vi "Autonomous Independent.vi"() -> ()   [LabVIEW 2015]
doc: "This VI is called when autonomous begins, and will automatically be terminated when autonomous ends. You can carry out timed or sensor driven robot movement independently without needing to return to the caller."
uses:
  <vilib>/Rock Robotics/WPI/CAN/TalonSRX/WPI_CANTalonSRX_BrakeOverride.ctl
  <vilib>/Rock Robotics/WPI/Solenoid/WPI_SolenoidValue.ctl
  <vilib>/Analysis/baseanly.llb/Mean (DBL).vi
  <vilib>/Rock Robotics/WPI/Utilities/WPI_GetSetVariantRefNum.vi
  <vilib>/Rock Robotics/Network Tables/NT Write Numeric Array.vi
  <vilib>/Rock Robotics/Network Tables/NT Read Numeric Array.vi
  <vilib>/Rock Robotics/Network Tables/NT Read String Array.vi
  <vilib>/Rock Robotics/Network Tables/NT Write String.vi
  <vilib>/addons/control/pid/pid.llb/PID (DBL).vi
  <vilib>/Rock Robotics/WPI/Solenoid/WPI_SolenoidSetEnum.vi
  ADI MXP IMU/ADI MXP IMU/FRC ADI MXP IMU.lvlib
  <vilib>/addons/control/pid/NI_PID_pid.lvlib
  <vilib>/Analysis/NI_AALBase.lvlib
panel:
  out "Waveform Chart":dbl(graph)
  out "Rotate PID Output":dbl(graph)
  # "Be sure to right-click and choose Data Operations>>Make Current Value default if you want to save the array values with the VI"
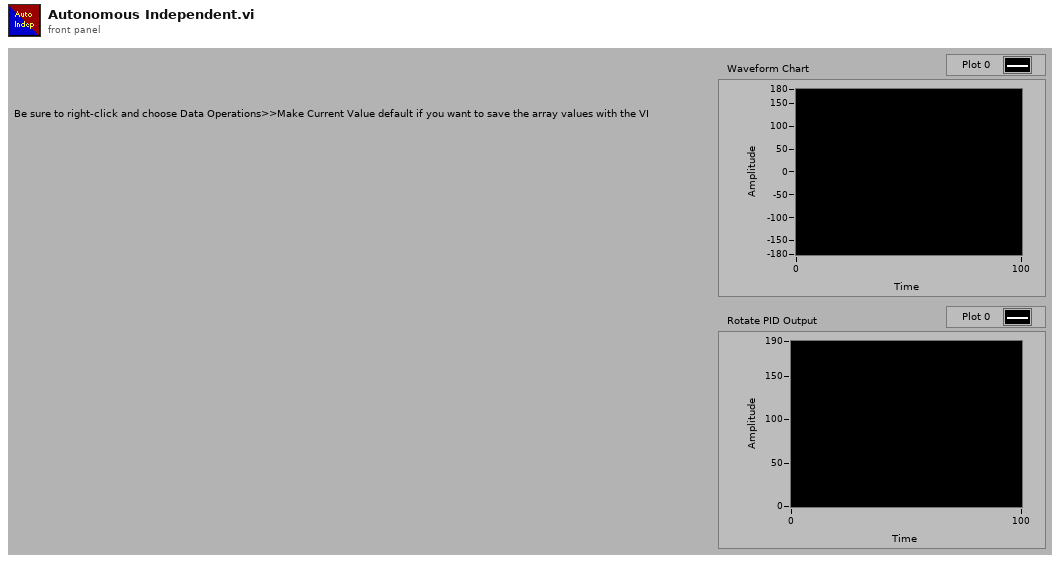
[diagram p1: front panel]
types:
  T1 = typedef "WPI_EncoderDevRef.ctl" = cluster{"DevStatus":errorcluster, "EncoderIndex":T2, "CounterIndex":T3, "DistancePerCount":dbl, "Decoding Type":T4}
  T2 = typedef "FPGA_EncoderIdx.ctl" = enum8{"Enc 0", "Enc 1", "Enc 2", "Enc 3", "Enc 4", "Enc 5", "Enc 6", "Enc 7", "Invalid"}
  T3 = typedef "FPGA_CounterCtrSystemIndex.ctl" = enum8{"Ctr 0", "Ctr 1", "Ctr 2", "Ctr 3", "Ctr 4", "Ctr 5", "Ctr 6", "Ctr 7", "Invalid"}
  T4 = typedef "WPI_EncoderType.ctl" = enum16{"1x", "2x", "4x"}
  T5 = cluster{"proportional gain (Kc)":dbl, "integral time (Ti, min)":dbl, "derivative time (Td, min)":dbl}
  T6 = typedef "WPI_SolenoidValue.ctl" = enum16{"Off", "On", "Forward", "Reverse"}
  T7 = typedef "WPI_CANTalonSRX_BrakeOverride.ctl" = enum8{"No Override", "Override to Coast", "Override to Brake"}
  T8 = typedef "FRC ADI MXP IMU.lvlib/WPI_AnalogDevicesIMUInterruptDevRef.ctl" = cluster{"SimpleGyroDevRef":T9, "InterruptRef":T11}
  T9 = typedef "FRC ADI MXP IMU.lvlib/WPI_AnalogDevicesIMUDevRef.ctl" = cluster{"DevStatus":errorcluster, "Handle":i32, "SPI Bus":T10, "Device Found":bool, "Sample Rate":dbl, "Device Ready":bool, "Yaw Axis":enum16{"X", "Y", "Z"}, "AHRS Algorithm":enum16{"Complementary", "Madgwick"}}
  T10 = typedef "spi_bus.ctl" = enum16{"SPI On-Board, CS0", "SPI On-Board, CS1", "SPI On-Board, CS2", "SPI On-Board, CS3", "SPI MXP", "Invalid"}
  T11 = typedef "WPI_InterruptRef.ctl" = cluster{"DevStatus":errorcluster, "InterruptIndex":T12}
  T12 = typedef "FPGA_InterruptIndex.ctl" = enum8{"0", "1", "2", "3", "4", "5", "6", "7", "Invalid"}
  T13 = typedef "WPI_SolenoidDevRef.ctl" = cluster{"DevStatus":errorcluster, "Pneumatics Control Module":u8, "Forward Solenoid Channel":T14, "Reverse Solenoid Channel":T14}
  T14 = typedef "WPI_SolenoidChannel.ctl" = enum8{"Solenoid 0", "Solenoid 1", "Solenoid 2", "Solenoid 3", "Solenoid 4", "Solenoid 5", "Solenoid 6", "Solenoid 7", "Invalid"}
  T15 = typedef "WPI_MotorControlDeviceRef.ctl" = cluster{"DeviceStatus":errorcluster, "Type":T16, "PWM":cluster{"PWM Channel":T17, "DeadBand":T18}, "CAN":cluster{"Device Number":u8, "Control Mode":T19, "Semaphore":T20, "Max Vout":dbl, "TalonSRX Control Mode":T21}, "Invert":bool}
  T16 = typedef "WPI_MotorControlType.ctl" = enum16{"PWM", "CAN", "CANTalonSRX"}
  T17 = typedef "FPGA_DIOPWMChannel.ctl" = enum8{"PWM 0", "PWM 1", "PWM 2", "PWM 3", "PWM 4", "PWM 5", "PWM 6", "PWM 7", "PWM 8", "PWM 9", "PWM MXP 0", "PWM MXP 1", "PWM MXP 2", "PWM MXP 3", "PWM MXP 4", "PWM MXP 5", "PWM MXP 6", "PWM MXP 7", "PWM MXP 8", "PWM MXP 9", "Invalid"}
  T18 = typedef "WPI_PWMDeadband.ctl" = cluster{"Name":string, "maxPositivePwm":i32, "minPositivePwm":i32, "centerPwm":i32, "maxNegativePwm":i32, "minNegativePwm":i32, "angularRange":u16}
  T19 = typedef "WPI_CANJaguar_ControlMode.ctl" = enum8{"Percent VBus", "Current", "Speed", "Position", "Voltage"}
  T20 = typedef "Semaphore RefNum" = refnum<k1>
  T21 = typedef "WPI_CANTalonSRX_APIControlMode.ctl" = enum8{"Percent VBus", "Speed", "Position", "Slave", "Unchanged / Invalid", "Voltage Compensation", "Current", "Motion Profile"}
  T22 = typedef "WPI_SwitchDevRef.ctl" = cluster{"DevStatus":errorcluster, "DIO Channel":T23, "CntIndex":T3, "Normally Closed":bool}
  T23 = typedef "FPGA_DIOChannel.ctl" = enum8{"DIO 0", "DIO 1", "DIO 2", "DIO 3", "DIO 4", "DIO 5", "DIO 6", "DIO 7", "DIO 8", "DIO 9", "DIO MXP 0", "DIO MXP 1", "DIO MXP 2", "DIO MXP 3", "DIO MXP 4", "DIO MXP 5", "DIO MXP 6", "DIO MXP 7", "DIO MXP 8", "DIO MXP 9", "DIO MXP 10", "DIO MXP 11", "DIO MXP 12", "DIO MXP 13", "DIO MXP 14", "DIO MXP 15", "Invalid"}
  T24 = cluster{"X Angle":dbl, "Y Angle":dbl, "Z Angle":dbl}
  T25 = typedef "WPI_JoystickDevRef.ctl" = cluster{"Device":T26}
  T26 = typedef "WPI_JoystickDeviceEnum.ctl" = enum16{"USB 0", "USB 1", "USB 2", "USB 3", "USB 4", "USB 5"}
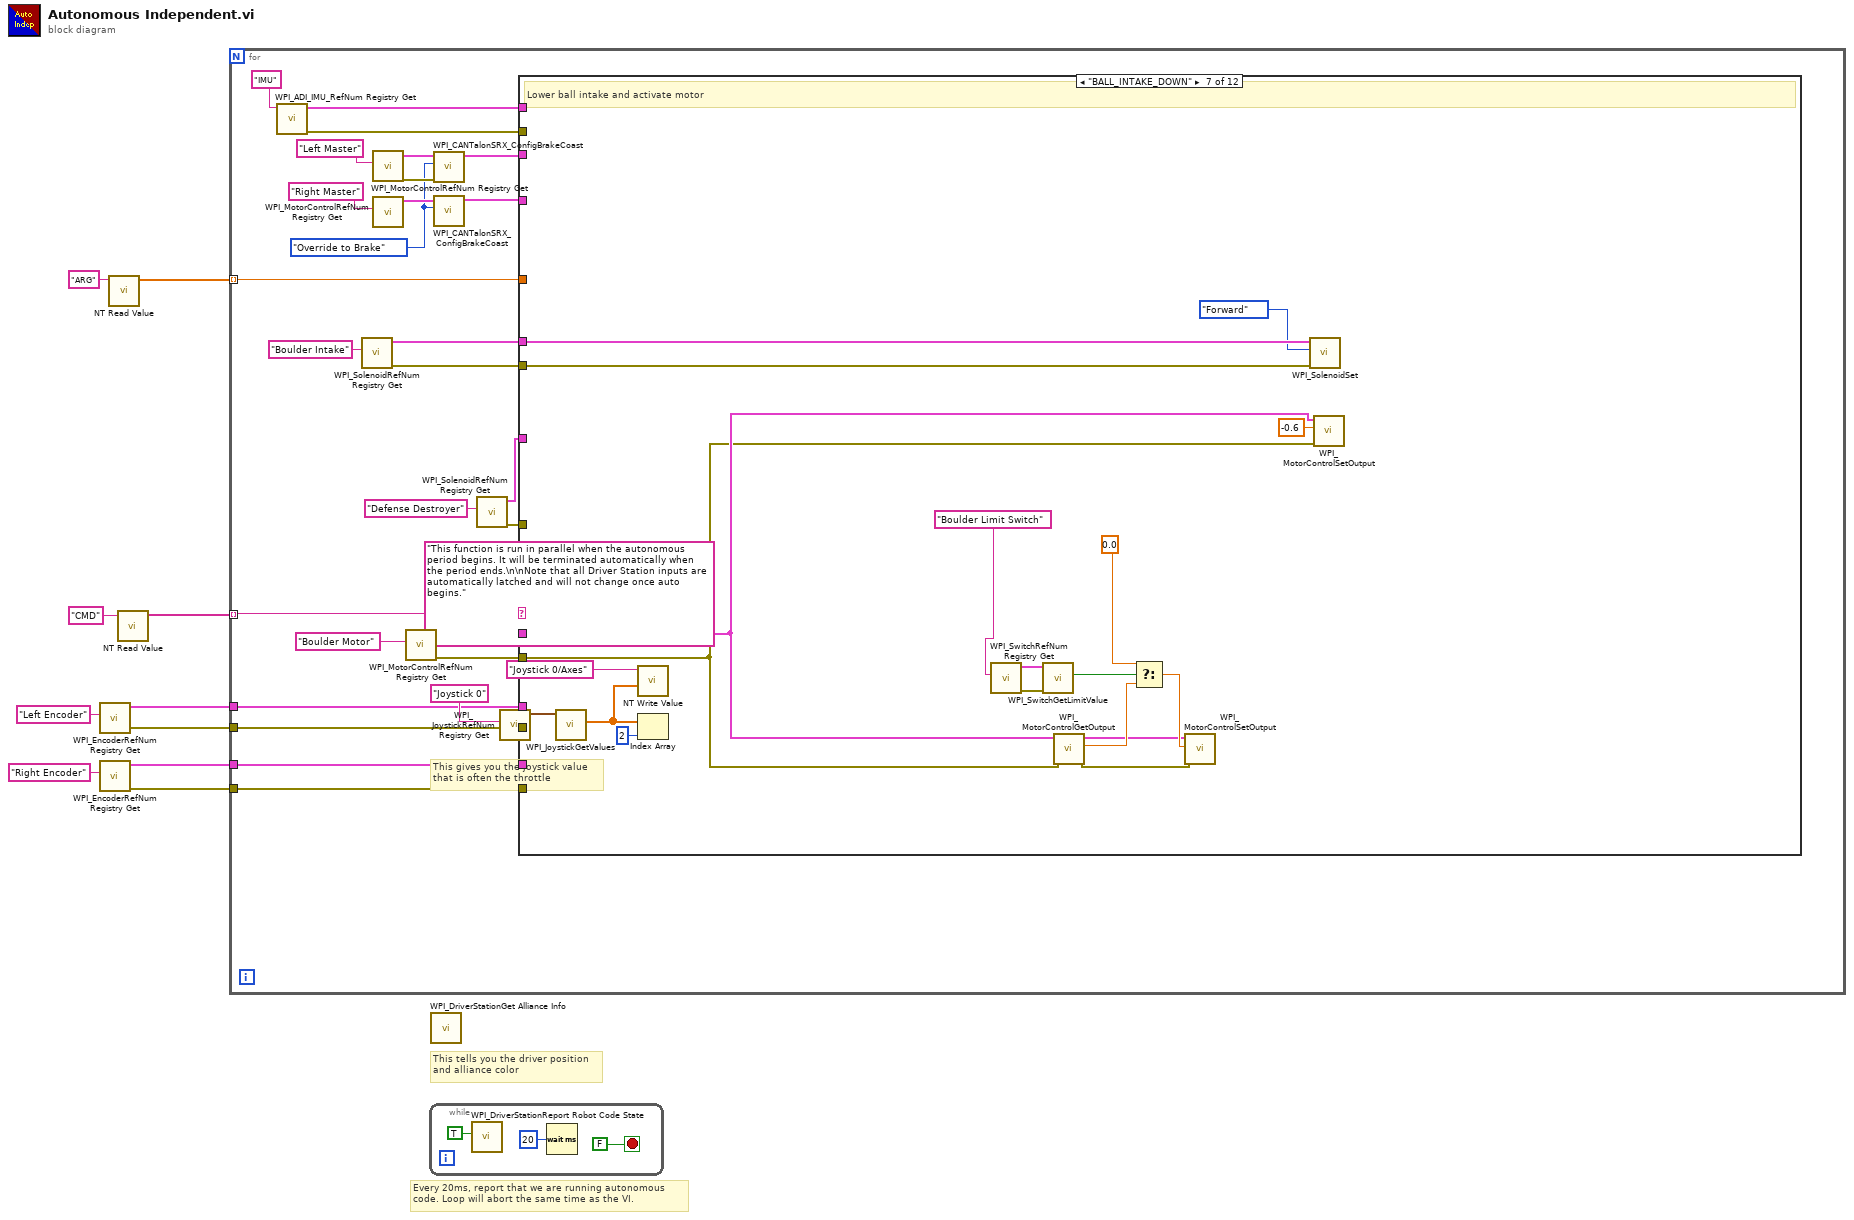
[diagram p0: block diagram]
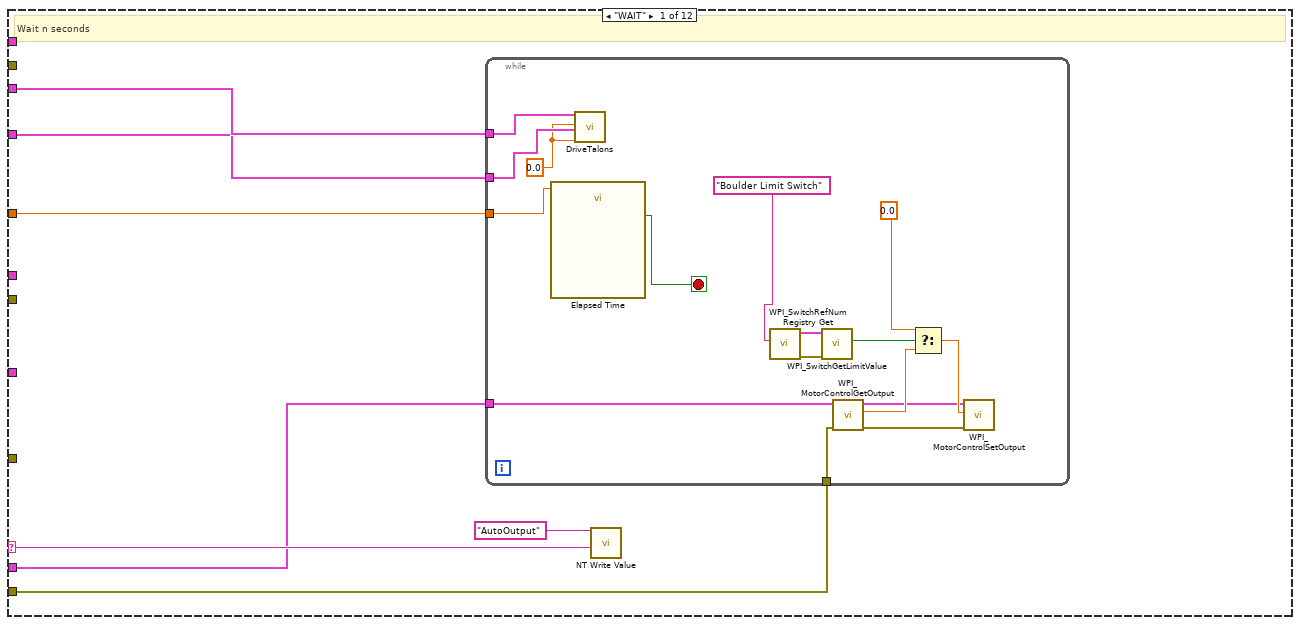
[diagram p2: hidden frame]
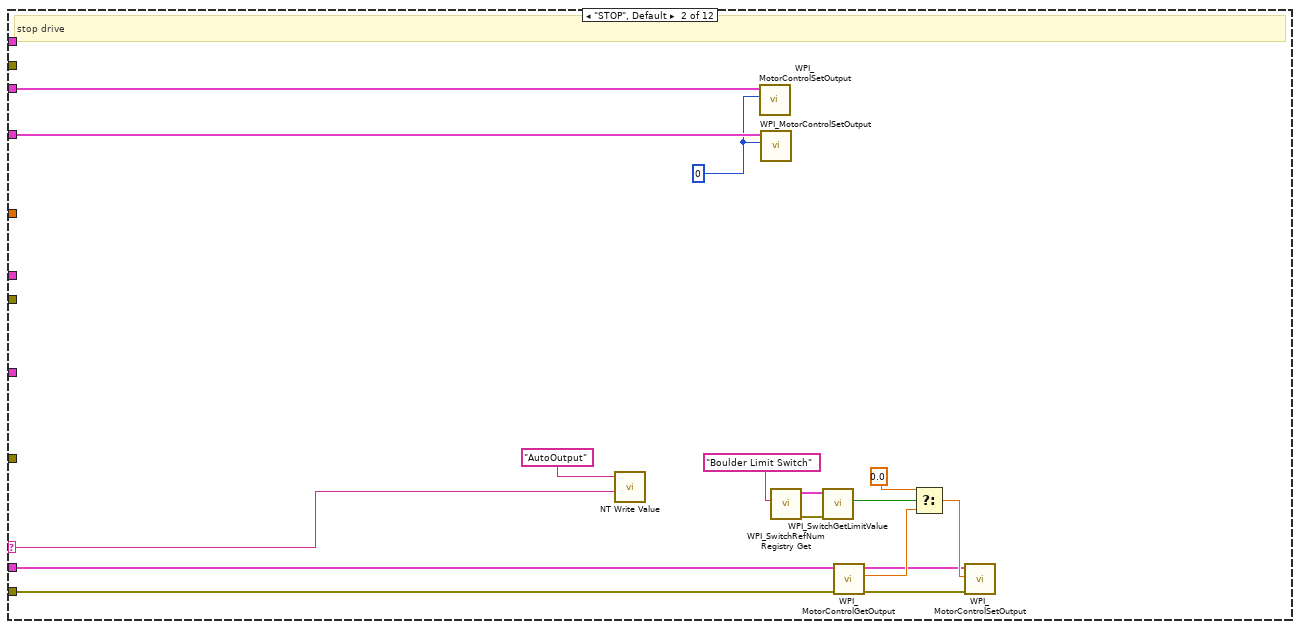
[diagram p3: hidden frame]
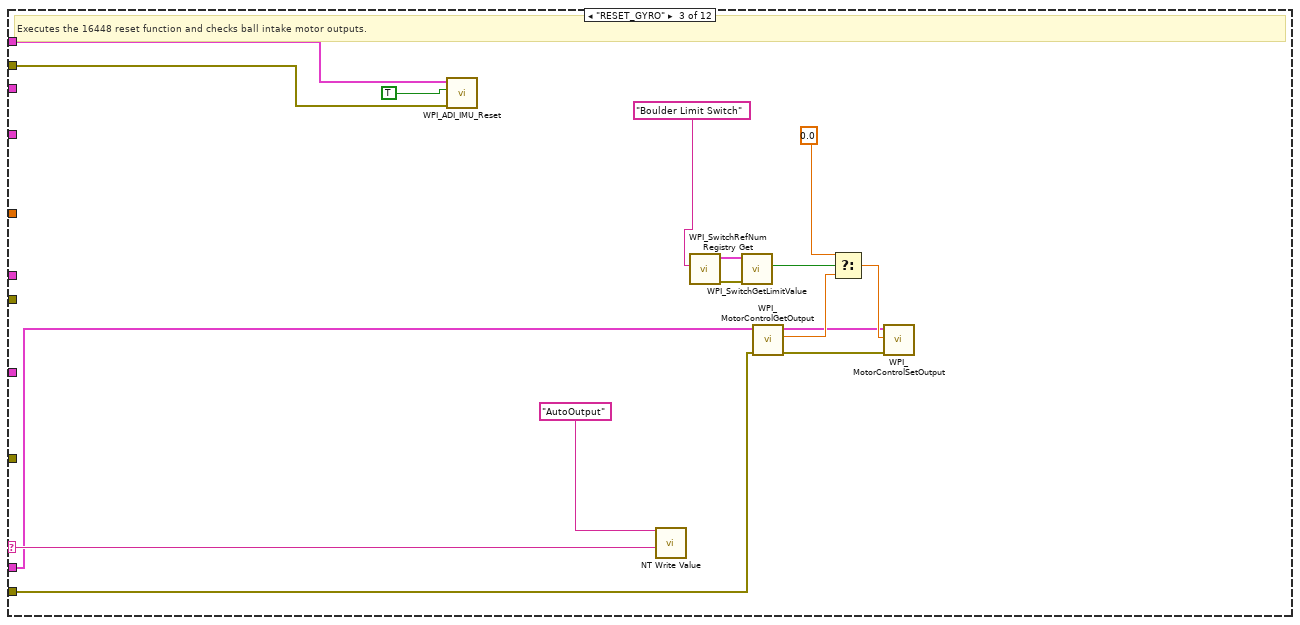
[diagram p4: hidden frame]
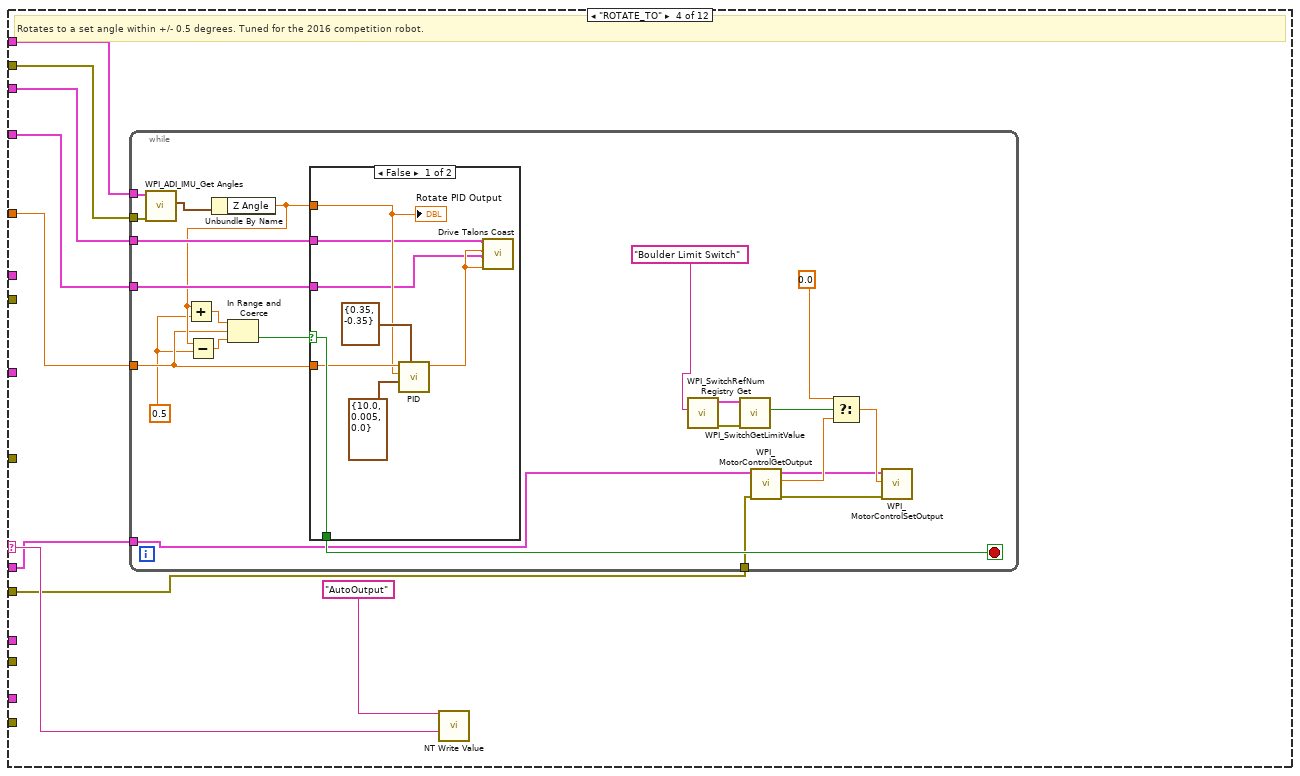
[diagram p5: hidden frame]
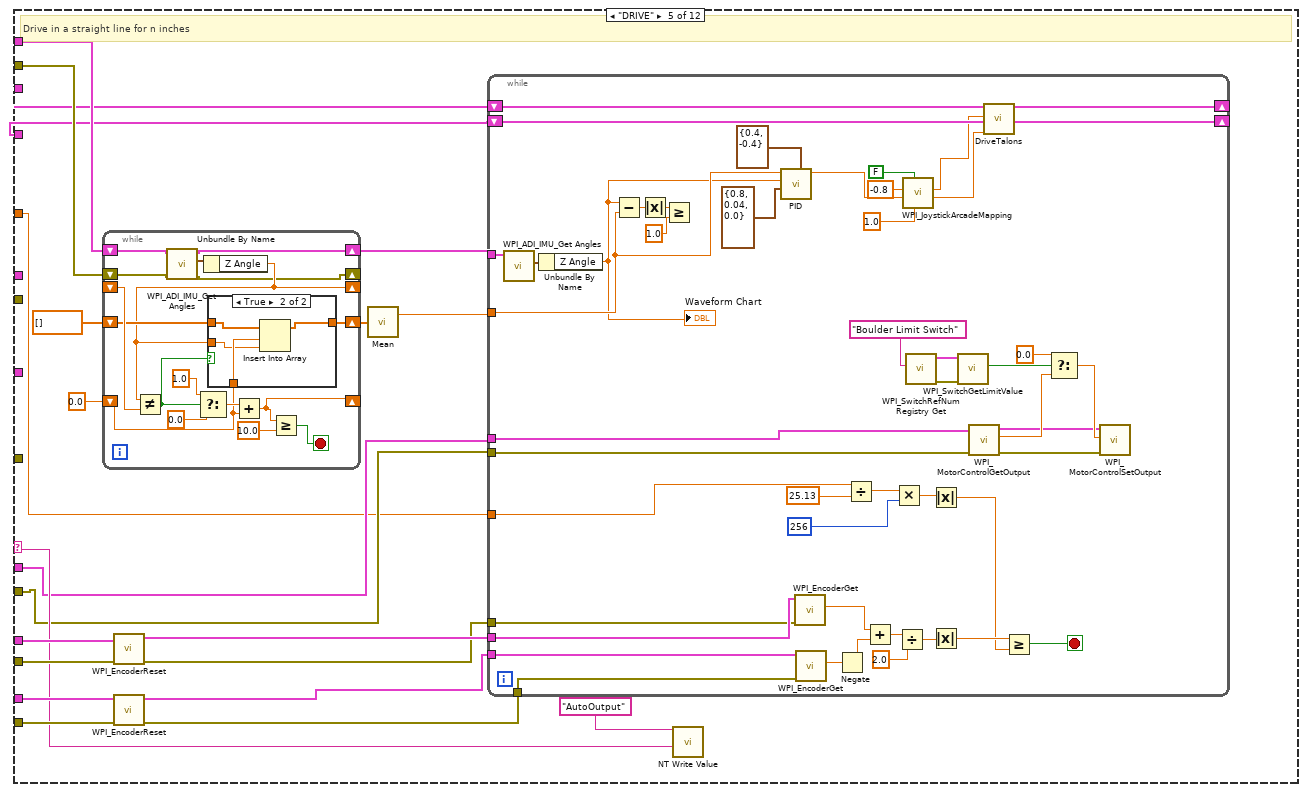
[diagram p7: hidden frame]
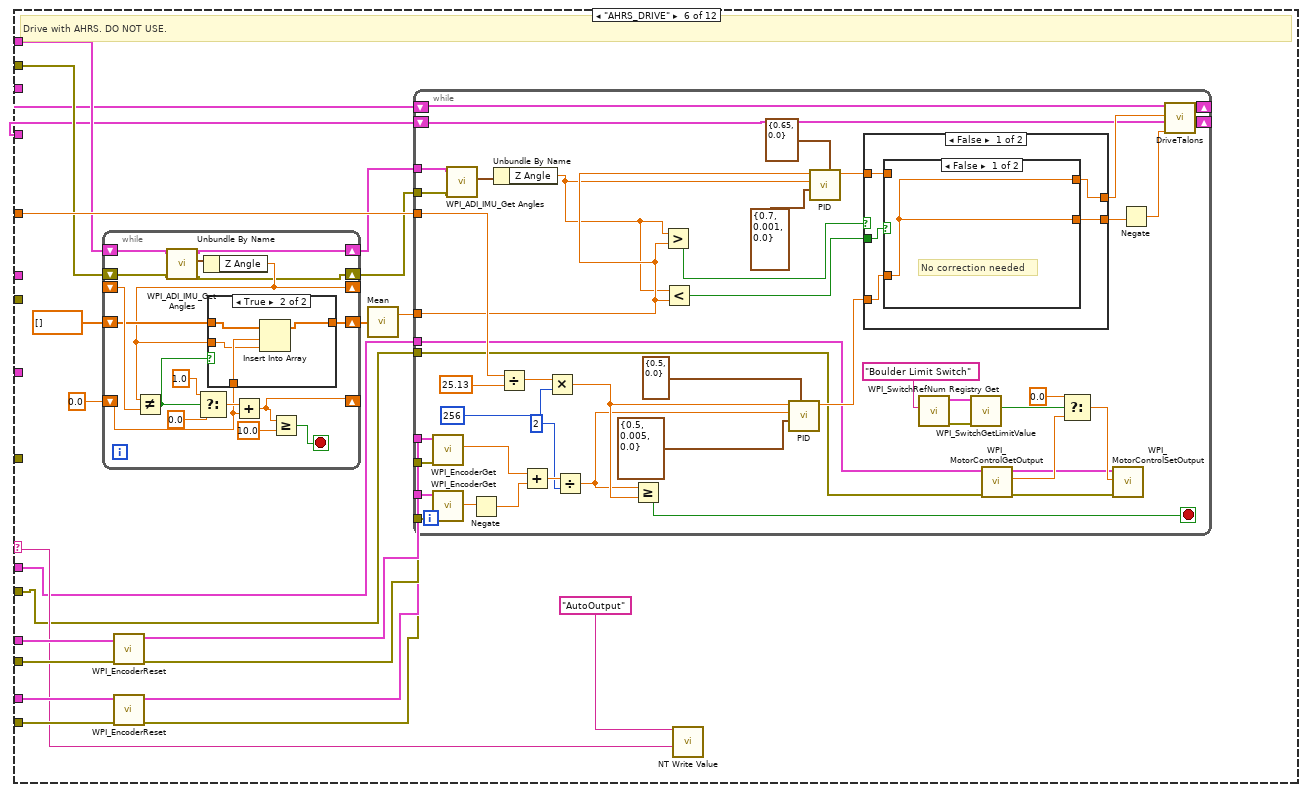
[diagram p9: hidden frame]
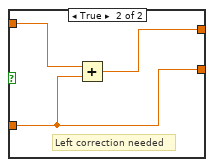
[diagram p11: hidden frame]
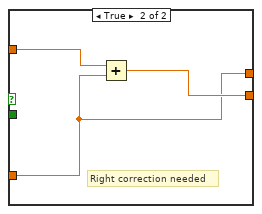
[diagram p12: hidden frame]
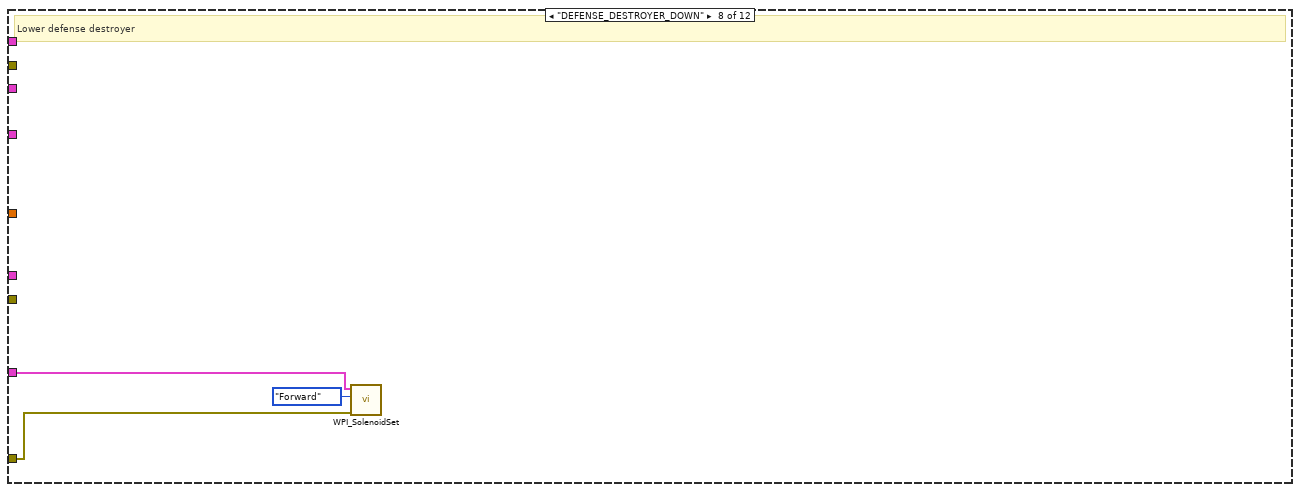
[diagram p13: hidden frame]
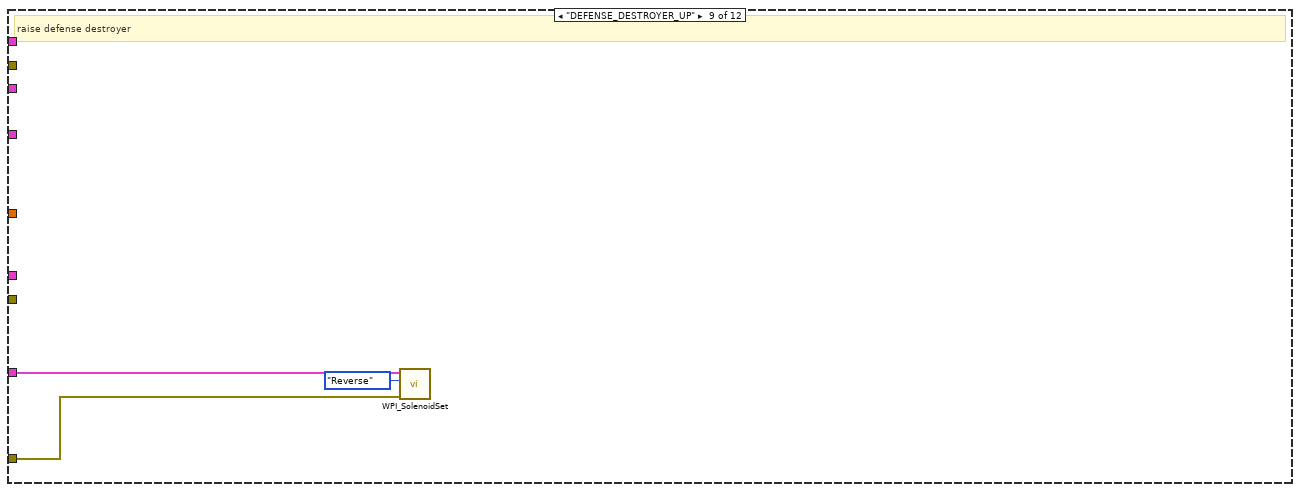
[diagram p14: hidden frame]
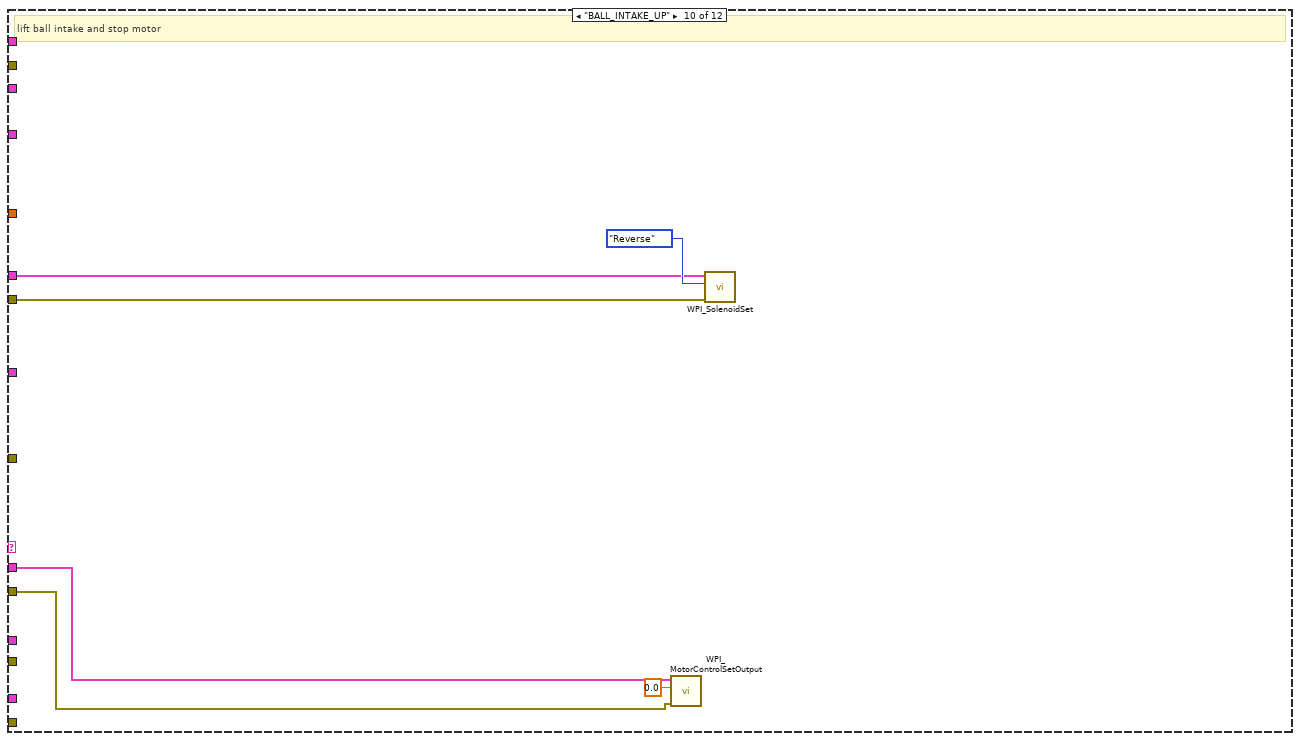
[diagram p15: hidden frame]
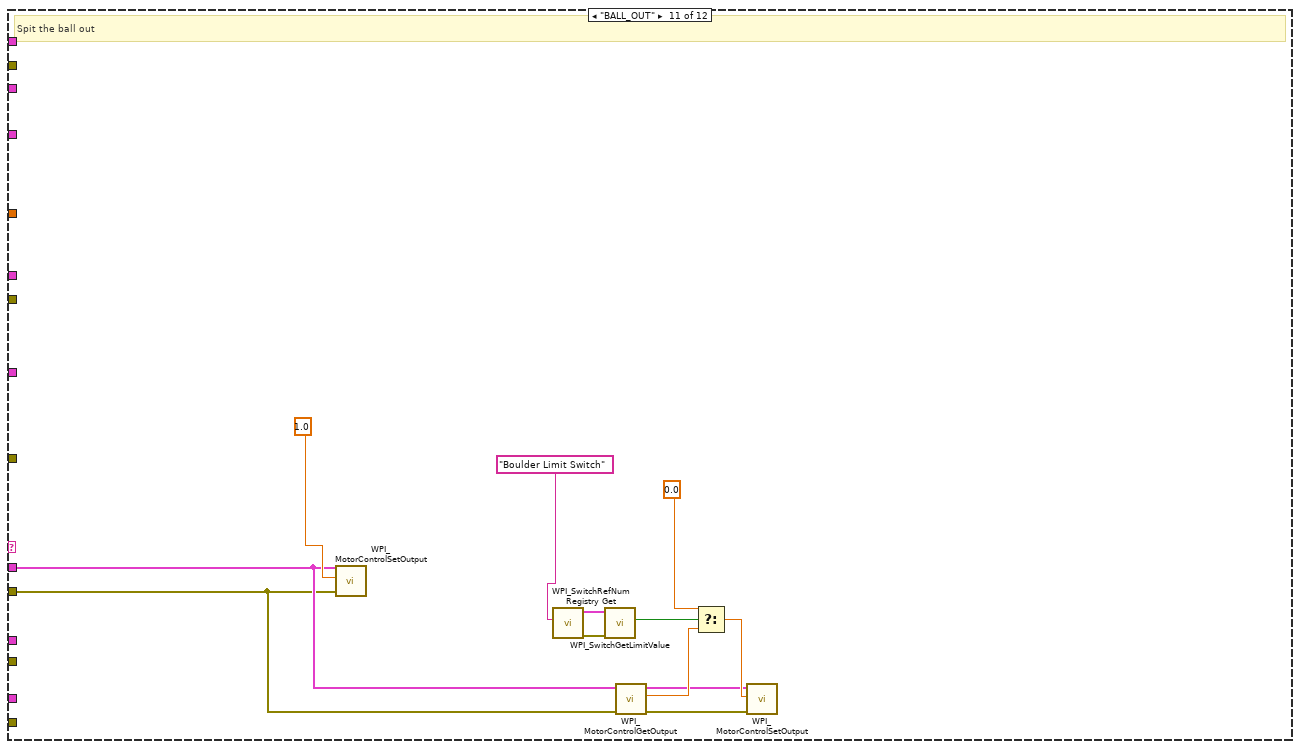
[diagram p16: hidden frame]
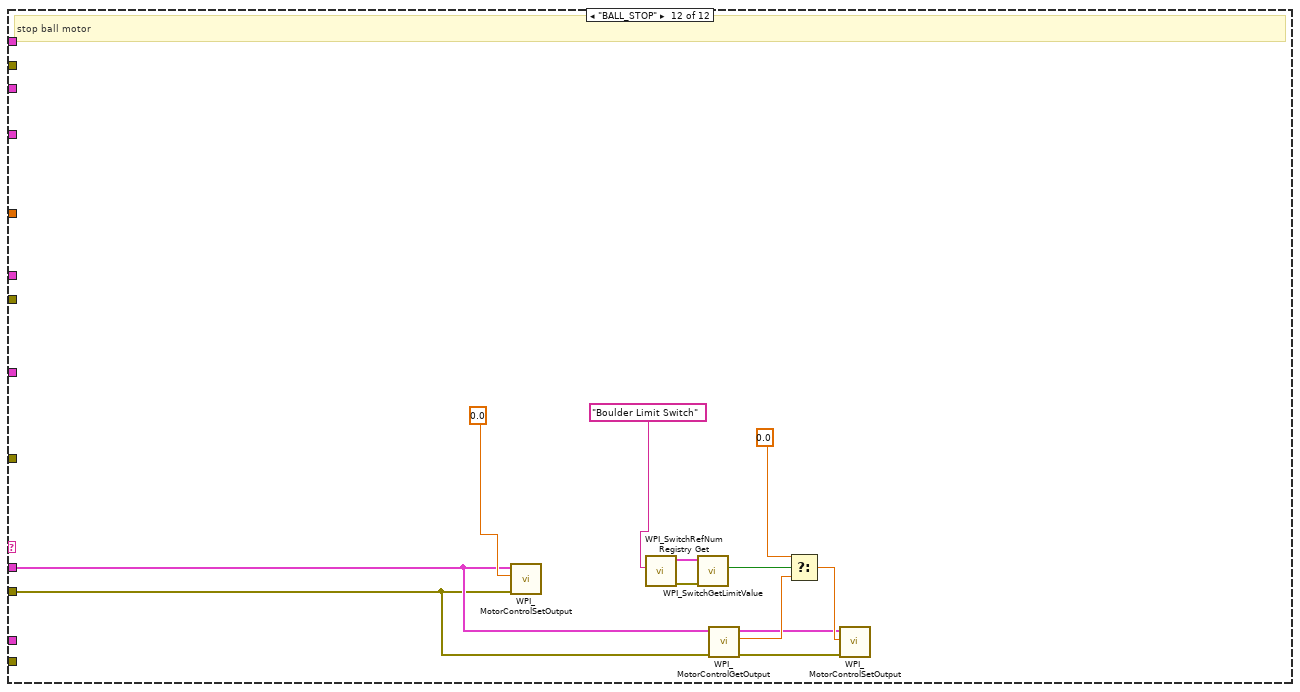
[diagram p17: hidden frame]
diagram:
  (unwired) "This function is run in parallel when the autonomous period begins. It will be terminated automatically when the period ends.\n\nNote that all Driver Station inputs are automatically latched and will not change once auto begins."
  # "Every 20ms, report that we are running autonomous\ncode. Loop will abort the same time as the VI."
  # "This gives you the joystick value\nthat is often the throttle"
  # "This tells you the driver position\nand alliance color"
  n1 = call <vilib>:"WPI_EncoderRefNum Registry Get.vi"("refnum name"="Left Encoder") -> ("error out"=w3:errorcluster, "EncoderDevRef"=w4:T1)  [unwired: 9 in]
  n2 = call <vilib>:"WPI_EncoderRefNum Registry Get.vi"("refnum name"="Right Encoder") -> ("error out"=w1:errorcluster, "EncoderDevRef"=w2:T1)  [unwired: 9 in]
  n3 = call-poly <vilib>:"NT Read Value.vi"("Name"="ARG") -> ("Numeric Array"=w8:dbl[])  [unwired: 9 in, 1 out]
  n4 = call-poly <vilib>:"NT Read Value.vi"("Name"="CMD") -> ("String Array"=w7:string[])  [unwired: 9 in, 1 out]
  n5 = for {
    tunnel: w7 -> [w41] mode=indexing
    tunnel: w8 -> [w40] mode=indexing
    tunnel: w4 -> [w37]
    tunnel: w3 -> [w36]
    tunnel: w2 -> [w35]
    tunnel: w1 -> [w34]
    w28 = WPI_CANTalonSRX_BrakeOverride."Override to Brake" ("Brake / Coast Mode")
    n6 = call "WPI_ADI_IMU_RefNum Registry Get.vi"("refnum name"="IMU") -> ("error out"=w19:errorcluster, "ADI IMU Interrupt DevRef"=w20:T8)  [unwired: 9 in]
    n7 = call <vilib>:"WPI_SolenoidRefNum Registry Get.vi"("refnum name"="Boulder Intake") -> ("error out"=w25:errorcluster, "SolenoidDevRef"=w26:T13)  [unwired: 9 in]
    n8 = call <vilib>:"WPI_MotorControlRefNum Registry Get.vi"("refnum name"="Left Master") -> ("error out"=w31:errorcluster, "MotorControlDevRef"=w32:T15)  [unwired: 9 in]
    n9 = call <vilib>:"WPI_MotorControlRefNum Registry Get.vi"("refnum name"="Right Master") -> ("MotorControlDevRef"=w30:T15)  [unwired: 9 in, 1 out]
    n10 = call <vilib>:"WPI_MotorControlRefNum Registry Get.vi"("refnum name"="Boulder Motor") -> ("error out"=w22:errorcluster, "MotorControlDevRef"=w23:T15)  [unwired: 9 in]
    n11 = call <vilib>:"WPI_CANTalonSRX_ConfigBrakeCoast.vi"("error in (no error)"=w31, "Brake / Coast Mode"=w28, "CAN Talon SRX Ref"=w32) -> ("CAN Talon SRX Ref"=w33:T15)  [unwired: 7 in, 1 out]
    n12 = call <vilib>:"WPI_CANTalonSRX_ConfigBrakeCoast.vi"("Brake / Coast Mode"=w28, "CAN Talon SRX Ref"=w30) -> ("CAN Talon SRX Ref"=w29:T15)  [unwired: 8 in, 1 out]
    n13 = call <vilib>:"WPI_SolenoidRefNum Registry Get.vi"("refnum name"="Defense Destroyer") -> ("error out"=w16:errorcluster, "SolenoidDevRef"=w17:T13)  [unwired: 9 in]
    n14 = case shown="\"BALL_INTAKE_DOWN\"" w41 {
      selector: w41 -> [w47 w79 w95 w101 w149 w232 _ _ _ _ _ _]
      tunnel: w33 -> [w45 w78 _ w100 w148 w236 _ _ _ _ _ _]
      tunnel: w40 -> [w46 _ _ w103 w142 w251 _ _ _ _ _ _]
      tunnel: w20 -> [_ _ w94 w105 w154 w242 _ _ _ _ _ _]
      tunnel: w19 -> [_ _ w93 w104 w153 w240 _ _ _ _ _ _]
      tunnel: w29 -> [w44 w77 _ w99 w147 w235 _ _ _ _ _ _]
      tunnel: w37 -> [_ _ _ _ w158 w250 _ _ _ _ _ _]
      tunnel: w36 -> [_ _ _ _ w157 w247 _ _ _ _ _ _]
      tunnel: w35 -> [_ _ _ _ w156 w246 _ _ _ _ _ _]
      tunnel: w34 -> [_ _ _ _ w155 w245 _ _ _ _ _ _]
      tunnel: w26 -> [_ _ _ _ _ _ w348 _ _ w359 _ _]
      tunnel: w25 -> [_ _ _ _ _ _ w347 _ _ w358 _ _]
      tunnel: w23 -> [w43 w66 w82 w98 w144 w231 w335 _ _ w357 w362 w374]
      tunnel: w22 -> [w42 w65 w81 w97 w143 w230 w334 _ _ w356 w361 w373]
      tunnel: w17 -> [_ _ _ _ _ _ _ w349 w354 _ _ _]
      tunnel: w16 -> [_ _ _ _ _ _ _ w350 w353 _ _ _]
      frame "WAIT" {
        # "Wait n seconds"
        n15 = while {
          tunnel: w46 -> [w64]
          tunnel: w45 -> [w62]
          tunnel: w44 -> [w61]
          tunnel: w43 -> [w50]
          tunnel: w42 -> [w49]
          stop <- w63 stop-if-true
          w60 = 0.0 ("Right Stick")
          n16 = call "Elapsed Time"("Time Target (s)"=w64) -> ("Time has Elapsed"=w63:bool)  [unwired: 11 in, 7 out]
          n17 = call "DriveTalons.vi"("Left Motor"=w62, "Left Stick"=w60, "Right Motor"=w61, "Right Stick"=w60) -> ()  [unwired: 12 in, 4 out]
          n18 = call <vilib>:"WPI_SwitchRefNum Registry Get.vi"("refnum name"="Boulder Limit Switch") -> ("error out"=w58:errorcluster, "SwitchDevRef"=w57:T22)  [unwired: 9 in]
          n19 = call <vilib>:"WPI_SwitchGetLimitValue.vi"("error in (no error)"=w58, "SwitchDevRef"=w57) -> ("Switch Pressed"=w56:bool)  [unwired: 7 in, 2 out]
          n20 = call <vilib>:"WPI_MotorControlGetOutput.vi"("error in (no error)"=w49, "MotorControlDevRef"=w50) -> ("error out"=w51:errorcluster, "Output"=w53:dbl, "MotorControlDevRef"=w52:T15)  [unwired: 7 in]
          n21 = Select(t=0.0, s=w56, f=w53) -> (s? t:f=w54:dbl)
          n22 = call <vilib>:"WPI_MotorControlSetOutput.vi"("error in (no error)"=w51, "Output"=w54, "MotorControlDevRef"=w52) -> ()  [unwired: 6 in, 3 out]
        }
        n23 = call-poly <vilib>:"NT Write Value.vi"("String"=w47, "Name"="AutoOutput") -> ()  [unwired: 9 in, 1 out]
      }
      frame "STOP", Default {
        w76 = 0
        # "stop drive"
        n24 = call-poly <vilib>:"NT Write Value.vi"("String"=w79, "Name"="AutoOutput") -> ()  [unwired: 9 in, 1 out]
        n25 = call <vilib>:"WPI_MotorControlSetOutput.vi"("Output"=w76, "MotorControlDevRef"=w78) -> ()  [unwired: 7 in, 3 out]
        n26 = call <vilib>:"WPI_MotorControlSetOutput.vi"("Output"=w76, "MotorControlDevRef"=w77) -> ()  [unwired: 7 in, 3 out]
        n27 = call <vilib>:"WPI_SwitchRefNum Registry Get.vi"("refnum name"="Boulder Limit Switch") -> ("error out"=w74:errorcluster, "SwitchDevRef"=w73:T22)  [unwired: 9 in]
        n28 = call <vilib>:"WPI_SwitchGetLimitValue.vi"("error in (no error)"=w74, "SwitchDevRef"=w73) -> ("Switch Pressed"=w72:bool)  [unwired: 7 in, 2 out]
        n29 = call <vilib>:"WPI_MotorControlGetOutput.vi"("error in (no error)"=w65, "MotorControlDevRef"=w66) -> ("error out"=w67:errorcluster, "Output"=w69:dbl, "MotorControlDevRef"=w68:T15)  [unwired: 7 in]
        n30 = Select(t=0.0, s=w72, f=w69) -> (s? t:f=w70:dbl)
        n31 = call <vilib>:"WPI_MotorControlSetOutput.vi"("error in (no error)"=w67, "Output"=w70, "MotorControlDevRef"=w68) -> ()  [unwired: 6 in, 3 out]
      }
      frame "RESET_GYRO" {
        # "Executes the 16448 reset function and checks ball intake motor outputs."
        n32 = call "WPI_ADI_IMU_Reset.vi"("error in"=w93, "Reset? (T)"=TRUE, "ADI IMU Interrupt DevRef"=w94) -> ()  [unwired: 7 in, 2 out]
        n33 = call-poly <vilib>:"NT Write Value.vi"("String"=w95, "Name"="AutoOutput") -> ()  [unwired: 9 in, 1 out]
        n34 = call <vilib>:"WPI_SwitchRefNum Registry Get.vi"("refnum name"="Boulder Limit Switch") -> ("error out"=w90:errorcluster, "SwitchDevRef"=w89:T22)  [unwired: 9 in]
        n35 = call <vilib>:"WPI_SwitchGetLimitValue.vi"("error in (no error)"=w90, "SwitchDevRef"=w89) -> ("Switch Pressed"=w88:bool)  [unwired: 7 in, 2 out]
        n36 = call <vilib>:"WPI_MotorControlGetOutput.vi"("error in (no error)"=w81, "MotorControlDevRef"=w82) -> ("error out"=w83:errorcluster, "Output"=w85:dbl, "MotorControlDevRef"=w84:T15)  [unwired: 7 in]
        n37 = Select(t=0.0, s=w88, f=w85) -> (s? t:f=w86:dbl)
        n38 = call <vilib>:"WPI_MotorControlSetOutput.vi"("error in (no error)"=w83, "Output"=w86, "MotorControlDevRef"=w84) -> ()  [unwired: 6 in, 3 out]
      }
      frame "ROTATE_TO" {
        # "Rotates to a set angle within +/- 0.5 degrees. Tuned for the 2016 competition robot."
        n39 = while {
          tunnel: w105 -> [w122]
          tunnel: w104 -> [w121]
          tunnel: w103 -> [w107]
          tunnel: w99 -> [w125]
          tunnel: w100 -> [w124]
          tunnel: w98 -> [w110]
          tunnel: w97 -> [w109]
          stop <- w128 stop-if-true
          w106 = 0.5 ("Within")
          n40 = call "WPI_ADI_IMU_Get Angles.vi"("error in"=w121, "ADI IMU Interrupt DevRef"=w122) -> ("IMU Angles"=w120:T24)  [unwired: 6 in, 3 out]
          n41 = Unbundle By Name(w120) -> ("Z Angle"=w123:dbl)
          n42 = Add(x=w123, y=w106) -> (x+y=w127:dbl)
          n43 = Subtract(x=w123, y=w106) -> (x-y=w126:dbl)
          n44 = In Range and Coerce(upper limit=w127, x=w107, lower limit=w126) -> (In Range?=w108:bool)  [unwired: 1 out]
          n45 = case shown="False" w108 {
            selector: w108 -> [w134 w137]
            tunnel: w107 -> [w133 _]
            tunnel: [w134 w137] -> w128
            tunnel: w123 -> [w132 _]
            tunnel: w125 -> [w129 _]
            tunnel: w124 -> [w131 _]
            frame False {
              n46 = call-poly <vilib>:"PID.vi"("output range"=cluster{"output high":dbl, "output low":dbl} {"output high"=0.35, "output low"=-0.35}, "PID gains"=T5 {"proportional gain (Kc)"=10.0, "integral time (Ti, min)"=0.005, "derivative time (Td, min)"=0.0}, "process variable"=w132, "setpoint"=w133) -> ("output"=w130:dbl)  [unwired: 6 in, 1 out]
              n47 = call "Drive Talons Coast.vi"("Left Motor"=w131, "Left Stick"=w130, "Right Motor"=w129, "Right Stick"=w130) -> ()  [unwired: 12 in, 4 out]
              "Rotate PID Output" <- w132
            }
            frame True {
            }
          }
          n48 = call <vilib>:"WPI_SwitchRefNum Registry Get.vi"("refnum name"="Boulder Limit Switch") -> ("error out"=w118:errorcluster, "SwitchDevRef"=w117:T22)  [unwired: 9 in]
          n49 = call <vilib>:"WPI_SwitchGetLimitValue.vi"("error in (no error)"=w118, "SwitchDevRef"=w117) -> ("Switch Pressed"=w116:bool)  [unwired: 7 in, 2 out]
          n50 = call <vilib>:"WPI_MotorControlGetOutput.vi"("error in (no error)"=w109, "MotorControlDevRef"=w110) -> ("error out"=w111:errorcluster, "Output"=w113:dbl, "MotorControlDevRef"=w112:T15)  [unwired: 7 in]
          n51 = Select(t=0.0, s=w116, f=w113) -> (s? t:f=w114:dbl)
          n52 = call <vilib>:"WPI_MotorControlSetOutput.vi"("error in (no error)"=w111, "Output"=w114, "MotorControlDevRef"=w112) -> ()  [unwired: 6 in, 3 out]
        }
        n53 = call-poly <vilib>:"NT Write Value.vi"("String"=w101, "Name"="AutoOutput") -> ()  [unwired: 9 in, 1 out]
      }
      frame "DRIVE" {
        # "Drive in a straight line for n inches"
        n54 = while {
          shift-right: [w215] -> _
          shift-left: _ -> [w224]
          shift-right: [w216] -> _
          shift-left: 0.0 -> [w213]
          shift-right: [w210] -> w146
          shift-left: w154 -> [w212]
          shift-right: [w209] -> _
          shift-left: w153 -> [w211]
          shift-right: [w214] -> w151
          shift-left: dbl[] [] -> [w217]
          stop <- w220 stop-if-true
          n55 = call "WPI_ADI_IMU_Get Angles.vi"("error in"=w211, "ADI IMU Interrupt DevRef"=w212) -> ("error out"=w209:errorcluster, "IMU Angles"=w208:T24, "ADI IMU Interrupt DevRef Out"=w210:T8)  [unwired: 6 in, 1 out]
          n56 = Unbundle By Name(w208) -> ("Z Angle"=w215:dbl)
          n57 = Not Equal?(x=w215, y=w224) -> (x != y?=w218:bool)
          n58 = Select(t=1.0, s=w218, f=0.0) -> (s? t:f=w221:dbl)
          n59 = case shown="True" w218 {
            tunnel: w217 -> [w225 w229]
            tunnel: [w225 w228] -> w214
            tunnel: w215 -> [_ w226]
            tunnel: w213 -> [_ w227]
            frame False {
            }
            frame True {
              n60 = Insert Into Array(array=w229, index=w227, new element=w226) -> (w228:dbl[])
            }
          }
          n61 = Add(x=w221, y=w213) -> (x+y=w216:dbl)
          n62 = Greater Or Equal?(x=w216, y=10.0) -> (x >= y?=w220:bool)
        }
        n63 = call <vilib>:"WPI_EncoderReset.vi"("error in (no error)"=w157, "EncoderDevRef"=w158) -> ("error out"=w140:errorcluster, "EncoderDevRef"=w141:T1)  [unwired: 8 in]
        n64 = call <vilib>:"WPI_EncoderReset.vi"("error in (no error)"=w155, "EncoderDevRef"=w156) -> ("error out"=w138:errorcluster, "EncoderDevRef"=w139:T1)  [unwired: 8 in]
        n65 = call-poly <vilib>:"Mean.vi"("X"=w151) -> ("mean"=w145:dbl)  [unwired: 1 out]
        n66 = while {
          tunnel: w146 -> [w198]
          tunnel: w145 -> [w203]
          shift-right: [w206] -> _
          shift-left: w147 -> [w205]
          shift-right: [w207] -> _
          shift-left: w148 -> [w204]
          tunnel: w144 -> [w187]
          tunnel: w143 -> [w186]
          tunnel: w142 -> [w179]
          tunnel: w141 -> [w169]
          tunnel: w140 -> [w168]
          tunnel: w139 -> [w167]
          tunnel: w138 -> [w166]
          stop <- w170 stop-if-true
          n67 = call "WPI_ADI_IMU_Get Angles.vi"("ADI IMU Interrupt DevRef"=w198) -> ("IMU Angles"=w197:T24)  [unwired: 7 in, 3 out]
          n68 = Unbundle By Name(w197) -> ("Z Angle"=w199:dbl)
          "Waveform Chart" <- w199
          n69 = Subtract(x=w199, y=w203) -> (x-y=w201:dbl)
          n70 = Absolute Value(x=w201) -> (abs(x)=w200:dbl)
          n71 = Greater Or Equal?(x=w200, y=1.0) -> ()  [unwired: 1 out]
          n72 = call-poly <vilib>:"PID.vi"("output range"=cluster{"output high":dbl, "output low":dbl} {"output high"=0.4, "output low"=-0.4}, "PID gains"=T5 {"proportional gain (Kc)"=0.8, "integral time (Ti, min)"=0.04, "derivative time (Td, min)"=0.0}, "process variable"=w199, "setpoint"=w203) -> ("output"=w172:dbl)  [unwired: 6 in, 1 out]
          n73 = call <vilib>:"WPI_EncoderGet.vi"("error in (no error)"=w168, "EncoderDevRef"=w169) -> ("Distance"=w185:dbl)  [unwired: 4 in, 5 out]
          n74 = call <vilib>:"WPI_EncoderGet.vi"("error in (no error)"=w166, "EncoderDevRef"=w167) -> ("Distance"=w165:dbl)  [unwired: 4 in, 5 out]
          n75 = Negate(x=w165) -> (-x=w164:dbl)
          n76 = Divide(x=w179, y=25.13) -> (x/y=w181:dbl)
          n77 = Add(x=w185, y=w164) -> (x+y=w184:dbl)
          n78 = Multiply(x=w181, y=256) -> (x*y=w161:dbl)
          n79 = Divide(x=w184, y=2.0) -> (x/y=w163:dbl)
          n80 = call <vilib>:"WPI_JoystickArcadeMapping.vi"("Max Output"=1.0, "Square Inputs"=FALSE, "Y axis value"=w172, "X axis value"=-0.8) -> ("Right Motor Value"=w173:dbl, "Left Motor Value"=w174:dbl)  [unwired: 6 in]
          n81 = call <vilib>:"WPI_SwitchRefNum Registry Get.vi"("refnum name"="Boulder Limit Switch") -> ("error out"=w195:errorcluster, "SwitchDevRef"=w194:T22)  [unwired: 9 in]
          n82 = Absolute Value(x=w161) -> (abs(x)=w160:dbl)
          n83 = Absolute Value(x=w163) -> (abs(x)=w162:dbl)
          n84 = call <vilib>:"WPI_SwitchGetLimitValue.vi"("error in (no error)"=w195, "SwitchDevRef"=w194) -> ("Switch Pressed"=w193:bool)  [unwired: 7 in, 2 out]
          n85 = call <vilib>:"WPI_MotorControlGetOutput.vi"("error in (no error)"=w186, "MotorControlDevRef"=w187) -> ("error out"=w188:errorcluster, "Output"=w190:dbl, "MotorControlDevRef"=w189:T15)  [unwired: 7 in]
          n86 = call "DriveTalons.vi"("Left Motor"=w204, "Left Stick"=w174, "Right Motor"=w205, "Right Stick"=w173) -> ("Left Motor Out"=w207:T15, "Right Motor Out"=w206:T15)  [unwired: 12 in, 2 out]
          n87 = Greater Or Equal?(x=w162, y=w160) -> (x >= y?=w170:bool)
          n88 = Select(t=0.0, s=w193, f=w190) -> (s? t:f=w191:dbl)
          n89 = call <vilib>:"WPI_MotorControlSetOutput.vi"("error in (no error)"=w188, "Output"=w191, "MotorControlDevRef"=w189) -> ()  [unwired: 6 in, 3 out]
        }
        n90 = call-poly <vilib>:"NT Write Value.vi"("String"=w149, "Name"="AutoOutput") -> ()  [unwired: 9 in, 1 out]
      }
      frame "AHRS_DRIVE" {
        # "Drive with AHRS. DO NOT USE."
        n91 = while {
          shift-right: [w260] -> _
          shift-left: _ -> [w269]
          shift-right: [w261] -> _
          shift-left: 0.0 -> [w258]
          shift-right: [w255] -> w241
          shift-left: w242 -> [w257]
          shift-right: [w254] -> w239
          shift-left: w240 -> [w256]
          shift-right: [w259] -> w237
          shift-left: dbl[] [] -> [w262]
          stop <- w265 stop-if-true
          n92 = call "WPI_ADI_IMU_Get Angles.vi"("error in"=w256, "ADI IMU Interrupt DevRef"=w257) -> ("error out"=w254:errorcluster, "IMU Angles"=w253:T24, "ADI IMU Interrupt DevRef Out"=w255:T8)  [unwired: 6 in, 1 out]
          n93 = Unbundle By Name(w253) -> ("Z Angle"=w260:dbl)
          n94 = Not Equal?(x=w260, y=w269) -> (x != y?=w263:bool)
          n95 = Select(t=1.0, s=w263, f=0.0) -> (s? t:f=w266:dbl)
          n96 = case shown="True" w263 {
            tunnel: w262 -> [w270 w274]
            tunnel: [w270 w273] -> w259
            tunnel: w260 -> [_ w271]
            tunnel: w258 -> [_ w272]
            frame False {
            }
            frame True {
              n97 = Insert Into Array(array=w274, index=w272, new element=w271) -> (w273:dbl[])
            }
          }
          n98 = Add(x=w266, y=w258) -> (x+y=w261:dbl)
          n99 = Greater Or Equal?(x=w261, y=10.0) -> (x >= y?=w265:bool)
        }
        n100 = call <vilib>:"WPI_EncoderReset.vi"("error in (no error)"=w247, "EncoderDevRef"=w250) -> ("error out"=w248:errorcluster, "EncoderDevRef"=w249:T1)  [unwired: 8 in]
        n101 = call <vilib>:"WPI_EncoderReset.vi"("error in (no error)"=w245, "EncoderDevRef"=w246) -> ("error out"=w243:errorcluster, "EncoderDevRef"=w244:T1)  [unwired: 8 in]
        n102 = call-poly <vilib>:"Mean.vi"("X"=w237) -> ("mean"=w233:dbl)  [unwired: 1 out]
        n103 = while {
          tunnel: w251 -> [w319]
          tunnel: w249 -> [w315]
          tunnel: w248 -> [w314]
          tunnel: w244 -> [w313]
          tunnel: w243 -> [w312]
          tunnel: w241 -> [w296]
          tunnel: w239 -> [w295]
          shift-right: [w287] -> _
          shift-left: w236 -> [w289]
          shift-right: [w286] -> _
          shift-left: w235 -> [w288]
          tunnel: w233 -> [w299]
          tunnel: w231 -> [w276]
          tunnel: w230 -> [w275]
          stop <- w311 stop-if-true
          n104 = call <vilib>:"WPI_EncoderGet.vi"("error in (no error)"=w314, "EncoderDevRef"=w315) -> ("Distance"=w306:dbl)  [unwired: 4 in, 5 out]
          n105 = call <vilib>:"WPI_EncoderGet.vi"("error in (no error)"=w312, "EncoderDevRef"=w313) -> ("Distance"=w304:dbl)  [unwired: 4 in, 5 out]
          n106 = call "WPI_ADI_IMU_Get Angles.vi"("error in"=w295, "ADI IMU Interrupt DevRef"=w296) -> ("IMU Angles"=w294:T24)  [unwired: 6 in, 3 out]
          n107 = Negate(x=w304) -> (-x=w305:dbl)
          n108 = Unbundle By Name(w294) -> ("Z Angle"=w297:dbl)
          n109 = Divide(x=w319, y=25.13) -> (x/y=w317:dbl)
          n110 = Add(x=w306, y=w305) -> (x+y=w321:dbl)
          n111 = Multiply(x=w317, y=256) -> (x*y=w310:dbl)
          n112 = Divide(x=w321, y=2) -> (x/y=w309:dbl)
          n113 = Greater Or Equal?(x=w309, y=w310) -> (x >= y?=w311:bool)
          n114 = Greater?(x=w297, y=w299) -> (0:w307:bool)
          n115 = Less?(x=w297, y=w299) -> (x < y?=w292:bool)
          n116 = call-poly <vilib>:"PID.vi"("output range"=cluster{"output high":dbl, "output low":dbl} {"output high"=0.5, "output low"=0.0}, "PID gains"=T5 {"proportional gain (Kc)"=0.5, "integral time (Ti, min)"=0.005, "derivative time (Td, min)"=0.0}, "process variable"=w309, "setpoint"=w310) -> ("output"=w308:dbl)  [unwired: 6 in, 1 out]
          n117 = call-poly <vilib>:"PID.vi"("output range"=cluster{"output high":dbl, "output low":dbl} {"output high"=0.65, "output low"=0.0}, "PID gains"=T5 {"proportional gain (Kc)"=0.7, "integral time (Ti, min)"=0.001, "derivative time (Td, min)"=0.0}, "process variable"=w297, "setpoint"=w299) -> ("output"=w298:dbl)  [unwired: 6 in, 1 out]
          n118 = case shown="False" w307 {
            tunnel: w298 -> [w326 w332]
            tunnel: [w322 w331] -> w290
            tunnel: [w324 w333] -> w293
            tunnel: w308 -> [w323 w331]
            tunnel: w292 -> [w325 _]
            frame False {
              n119 = case shown="False" w325 {
                tunnel: [w327 w330] -> w322
                tunnel: w326 -> [_ w329]
                tunnel: [w327 w328] -> w324
                tunnel: w323 -> [w327 w328]
                frame False {
                  # "No correction needed"
                }
                frame True {
                  # "Left correction needed"
                  n120 = Add(x=w329, y=w328) -> (x+y=w330:dbl)
                }
              }
            }
            frame True {
              # "Right correction needed"
              n121 = Add(x=w332, y=w331) -> (x+y=w333:dbl)
            }
          }
          n122 = call <vilib>:"WPI_SwitchRefNum Registry Get.vi"("refnum name"="Boulder Limit Switch") -> ("error out"=w284:errorcluster, "SwitchDevRef"=w283:T22)  [unwired: 9 in]
          n123 = call <vilib>:"WPI_SwitchGetLimitValue.vi"("error in (no error)"=w284, "SwitchDevRef"=w283) -> ("Switch Pressed"=w282:bool)  [unwired: 7 in, 2 out]
          n124 = call <vilib>:"WPI_MotorControlGetOutput.vi"("error in (no error)"=w275, "MotorControlDevRef"=w276) -> ("error out"=w277:errorcluster, "Output"=w279:dbl, "MotorControlDevRef"=w278:T15)  [unwired: 7 in]
          n125 = Select(t=0.0, s=w282, f=w279) -> (s? t:f=w280:dbl)
          n126 = call <vilib>:"WPI_MotorControlSetOutput.vi"("error in (no error)"=w277, "Output"=w280, "MotorControlDevRef"=w278) -> ()  [unwired: 6 in, 3 out]
          n127 = Negate(x=w293) -> (-x=w291:dbl)
          n128 = call "DriveTalons.vi"("Left Motor"=w289, "Left Stick"=w290, "Right Motor"=w288, "Right Stick"=w291) -> ("Left Motor Out"=w287:T15, "Right Motor Out"=w286:T15)  [unwired: 12 in, 2 out]
        }
        n129 = call-poly <vilib>:"NT Write Value.vi"("String"=w232, "Name"="AutoOutput") -> ()  [unwired: 9 in, 1 out]
      }
      frame "BALL_INTAKE_DOWN" {
        # "Lower ball intake and activate motor"
        n130 = call <vilib>:"WPI_SwitchRefNum Registry Get.vi"("refnum name"="Boulder Limit Switch") -> ("error out"=w344:errorcluster, "SwitchDevRef"=w343:T22)  [unwired: 9 in]
        n131 = call <vilib>:"WPI_SwitchGetLimitValue.vi"("error in (no error)"=w344, "SwitchDevRef"=w343) -> ("Switch Pressed"=w342:bool)  [unwired: 7 in, 2 out]
        n132 = call <vilib>:"WPI_MotorControlGetOutput.vi"("error in (no error)"=w334, "MotorControlDevRef"=w335) -> ("error out"=w337:errorcluster, "Output"=w339:dbl, "MotorControlDevRef"=w338:T15)  [unwired: 7 in]
        n133 = Select(t=0.0, s=w342, f=w339) -> (s? t:f=w340:dbl)
        n134 = call <vilib>:"WPI_MotorControlSetOutput.vi"("error in (no error)"=w337, "Output"=w340, "MotorControlDevRef"=w338) -> ()  [unwired: 6 in, 3 out]
        n135 = call-poly <vilib>:"WPI_SolenoidSet.vi"("error in (no error)"=w347, "Value"=WPI_SolenoidValue."Forward", "SolenoidDevRef"=w348) -> ()  [unwired: 7 in, 2 out]
        n136 = call <vilib>:"WPI_MotorControlSetOutput.vi"("error in (no error)"=w334, "Output"=-0.6, "MotorControlDevRef"=w335) -> ()  [unwired: 6 in, 3 out]
      }
      frame "DEFENSE_DESTROYER_DOWN" {
        # "Lower defense destroyer"
        n137 = call-poly <vilib>:"WPI_SolenoidSet.vi"("error in (no error)"=w350, "Value"=WPI_SolenoidValue."Forward", "SolenoidDevRef"=w349) -> ()  [unwired: 7 in, 2 out]
      }
      frame "DEFENSE_DESTROYER_UP" {
        # "raise defense destroyer"
        n138 = call-poly <vilib>:"WPI_SolenoidSet.vi"("error in (no error)"=w353, "Value"=WPI_SolenoidValue."Reverse", "SolenoidDevRef"=w354) -> ()  [unwired: 7 in, 2 out]
      }
      frame "BALL_INTAKE_UP" {
        # "lift ball intake and stop motor"
        n139 = call <vilib>:"WPI_MotorControlSetOutput.vi"("error in (no error)"=w356, "Output"=0.0, "MotorControlDevRef"=w357) -> ()  [unwired: 6 in, 3 out]
        n140 = call-poly <vilib>:"WPI_SolenoidSet.vi"("error in (no error)"=w358, "Value"=WPI_SolenoidValue."Reverse", "SolenoidDevRef"=w359) -> ()  [unwired: 7 in, 2 out]
      }
      frame "BALL_OUT" {
        # "Spit the ball out"
        n141 = call <vilib>:"WPI_MotorControlSetOutput.vi"("error in (no error)"=w361, "Output"=1.0, "MotorControlDevRef"=w362) -> ()  [unwired: 6 in, 3 out]
        n142 = call <vilib>:"WPI_SwitchRefNum Registry Get.vi"("refnum name"="Boulder Limit Switch") -> ("error out"=w370:errorcluster, "SwitchDevRef"=w369:T22)  [unwired: 9 in]
        n143 = call <vilib>:"WPI_SwitchGetLimitValue.vi"("error in (no error)"=w370, "SwitchDevRef"=w369) -> ("Switch Pressed"=w368:bool)  [unwired: 7 in, 2 out]
        n144 = call <vilib>:"WPI_MotorControlGetOutput.vi"("error in (no error)"=w361, "MotorControlDevRef"=w362) -> ("error out"=w363:errorcluster, "Output"=w365:dbl, "MotorControlDevRef"=w364:T15)  [unwired: 7 in]
        n145 = Select(t=0.0, s=w368, f=w365) -> (s? t:f=w366:dbl)
        n146 = call <vilib>:"WPI_MotorControlSetOutput.vi"("error in (no error)"=w363, "Output"=w366, "MotorControlDevRef"=w364) -> ()  [unwired: 6 in, 3 out]
      }
      frame "BALL_STOP" {
        # "stop ball motor"
        n147 = call <vilib>:"WPI_MotorControlSetOutput.vi"("error in (no error)"=w373, "Output"=0.0, "MotorControlDevRef"=w374) -> ()  [unwired: 6 in, 3 out]
        n148 = call <vilib>:"WPI_SwitchRefNum Registry Get.vi"("refnum name"="Boulder Limit Switch") -> ("error out"=w382:errorcluster, "SwitchDevRef"=w381:T22)  [unwired: 9 in]
        n149 = call <vilib>:"WPI_SwitchGetLimitValue.vi"("error in (no error)"=w382, "SwitchDevRef"=w381) -> ("Switch Pressed"=w380:bool)  [unwired: 7 in, 2 out]
        n150 = call <vilib>:"WPI_MotorControlGetOutput.vi"("error in (no error)"=w373, "MotorControlDevRef"=w374) -> ("error out"=w375:errorcluster, "Output"=w377:dbl, "MotorControlDevRef"=w376:T15)  [unwired: 7 in]
        n151 = Select(t=0.0, s=w380, f=w377) -> (s? t:f=w378:dbl)
        n152 = call <vilib>:"WPI_MotorControlSetOutput.vi"("error in (no error)"=w375, "Output"=w378, "MotorControlDevRef"=w376) -> ()  [unwired: 6 in, 3 out]
      }
    }
  }
  n153 = while {
    stop <- FALSE stop-if-true
    n154 = call <vilib>:"WPI_DriverStationReport Robot Code State.vi"("Autonomous"=TRUE) -> ()  [unwired: 10 in, 1 out]
    n155 = Wait (ms)(milliseconds to wait=u32 20) -> ()  [unwired: 1 out]
  }
  n156 = call <vilib>:"WPI_DriverStationGet Alliance Info.vi"() -> ()  [unwired: 12 out]
  n157 = call <vilib>:"WPI_JoystickRefNum Registry Get.vi"("refnum name"="Joystick 0") -> ("JoystickDevRef"=w14:T25)  [unwired: 1 in, 9 out]
  n158 = call <vilib>:"WPI_JoystickGetValues.vi"("JoystickDevRef"=w14) -> ("Axes"=w12:dbl[])  [unwired: 6 in, 4 out]
  n159 = call-poly <vilib>:"NT Write Value.vi"("Numeric Array"=w12, "Name"="Joystick 0/Axes") -> ()  [unwired: 9 in, 1 out]
  n160 = Index Array(array=w12, index=2) -> ()  [unwired: 1 out]
